vi "Test Assert Equal.vi"(8 "error in (no error)":errorcluster) -> (0 "error out":errorcluster)   [LabVIEW 2009]
uses:
  classes/Assert/Assert.lvclass
  classes/Test/Test.lvclass
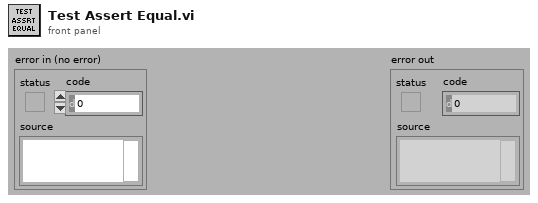
[diagram p1: front panel]
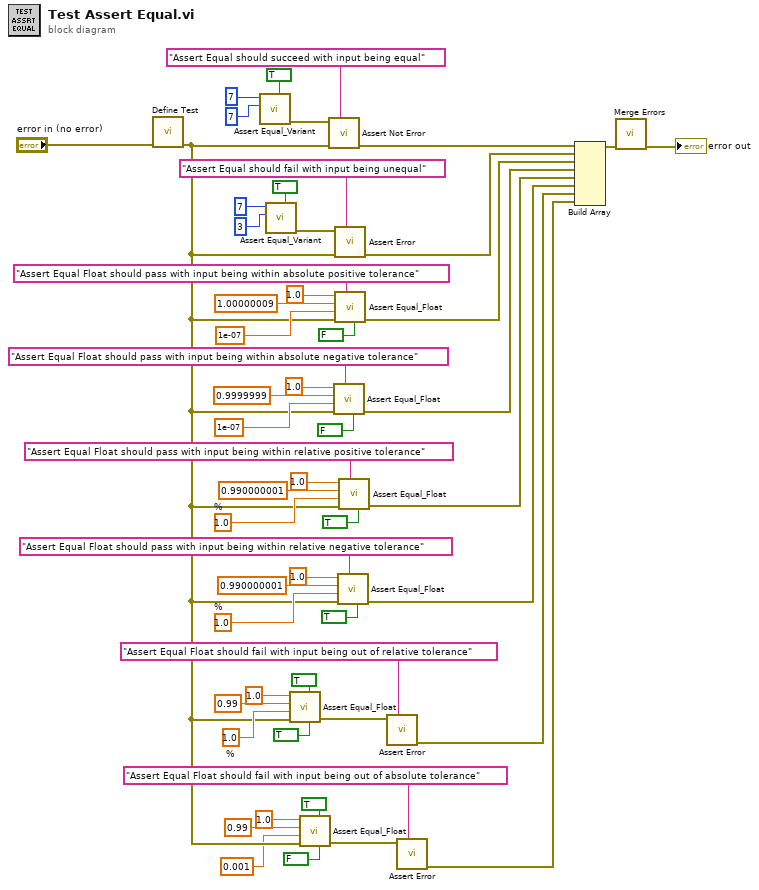
[diagram p0: block diagram]
diagram:
  w13 = 1.0  # %
  w20 = 1.0  # %
  w25 = 1.0  # %
  n1 = call "Define Test.vi"("error in (no error)"="error in (no error)") -> ("error out"=w3:errorcluster)  [unwired: 10 in]
  n2 = call "Assert Equal_Variant.vi"("Assert Only? (F)"=TRUE, "Y"=7, "X"=7) -> ("error out"=w56:errorcluster)  [unwired: 8 in]
  n3 = call "Assert Equal_Variant.vi"("Assert Only? (F)"=TRUE, "Y"=3, "X"=7) -> ("error out"=w54:errorcluster)  [unwired: 8 in]
  n4 = call "Assert Equal_Float.vi"("Use Percentage of X (F)"=TRUE, "Assert Only? (F)"=TRUE, "error in (no error)"=w3, "Tolerance"=w13, "Y"=0.99, "X"=1.0) -> ("error out"=w11:errorcluster)  [unwired: 5 in]
  n5 = call "Assert Equal_Float.vi"("Use Percentage of X (F)"=FALSE, "Assert Only? (F)"=TRUE, "error in (no error)"=w3, "Tolerance"=0.001, "Y"=0.99, "X"=1.0) -> ("error out"=w9:errorcluster)  [unwired: 5 in]
  n6 = call "Assert Not Error.vi"("Label"="Assert Equal should succeed with input being equal", "error in (no error)"=w3, "Not Error?"=w56) -> ("error out"=w44:errorcluster)  [unwired: 8 in]
  n7 = call "Assert Equal_Float.vi"("Use Percentage of X (F)"=FALSE, "Label"="Assert Equal Float should pass with input being within absolute negative tolerance", "error in (no error)"=w3, "Tolerance"=1e-07, "Y"=0.9999999, "X"=1.0) -> ("error out"=w30:errorcluster)  [unwired: 5 in]
  n8 = call "Assert Error.vi"("Label"="Assert Equal should fail with input being unequal", "error in (no error)"=w3, "Error?"=w54) -> ("error out"=w43:errorcluster)  [unwired: 8 in]
  n9 = call "Assert Equal_Float.vi"("Use Percentage of X (F)"=FALSE, "Label"="Assert Equal Float should pass with input being within absolute positive tolerance", "error in (no error)"=w3, "Tolerance"=1e-07, "Y"=1.00000009, "X"=1.0) -> ("error out"=w40:errorcluster)  [unwired: 5 in]
  n10 = call "Assert Equal_Float.vi"("Use Percentage of X (F)"=TRUE, "Label"="Assert Equal Float should pass with input being within relative negative tolerance", "error in (no error)"=w3, "Tolerance"=w20, "Y"=0.990000001, "X"=1.0) -> ("error out"=w18:errorcluster)  [unwired: 5 in]
  n11 = call "Assert Equal_Float.vi"("Use Percentage of X (F)"=TRUE, "Label"="Assert Equal Float should pass with input being within relative positive tolerance", "error in (no error)"=w3, "Tolerance"=w25, "Y"=0.990000001, "X"=1.0) -> ("error out"=w19:errorcluster)  [unwired: 5 in]
  n12 = call "Assert Error.vi"("Label"="Assert Equal Float should fail with input being out of relative tolerance", "Error?"=w11) -> ("error out"=w10:errorcluster)  [unwired: 9 in]
  n13 = call "Assert Error.vi"("Label"="Assert Equal Float should fail with input being out of absolute tolerance", "Error?"=w9) -> ("error out"=w1:errorcluster)  [unwired: 9 in]
  n14 = Build Array(w44, w43, w40, w30, w19, w18, w10, w1) -> (w42:errorcluster[])
  n15 = call <vilib>:"Merge Errors.vi"("error array in"=w42) -> ("error out"=→"error out":errorcluster)  [unwired: 6 in]
